vi "1_SimpleDemo_MHHisto.vi"() -> ()   [LabVIEW 2010]
uses:
  _lib/PQ/MultiHarp/mhlib_x86_x64_UIThread.llb/MH_DllPath_global.vi
  _lib/PQ/MultiHarp/MH_RefSource.ctl
  _lib/PQ/MultiHarp/MH_LibVersion_global.vi
  _lib/PQ/MultiHarp/MH_MeasMode.ctl
panel:
  in  "EnableInputDeadTime":bool caption="Enable DeadTime"
  in  "InputDeadTime":i32=1000 caption="DeadTime [ps]" min=800 max=160000 step=1
  in  "Trg.Edge":i32(ring) items=["falling", "rising"]
  in  "Trg.Level":i32=-100 caption="Trg.Level [mV]" min=-1200 max=1200 step=1
  in  "Offset":i32 caption="Offset [ps]" min=-99999 max=99999 step=1
  in  "Enable":bool=TRUE
  in  "EnableSyncDeadTime":bool caption="Enable DeadTime"
  in  "SyncDeadTime":i32=1000 caption="SyncDeadTime [ps]" min=800 max=160000 step=1
  in  "SyncTrg.Edge":i32(ring) items=["falling", "rising"]
  in  "SyncTrg.Level":i32=-100 caption="SyncTrg.Level [mV]" min=-1200 max=1200 step=1
  in  "SyncOffset":i32 caption="SyncOffset [ps]" min=-99999 max=99999 step=1
  in  "SyncDivider":i32(ring)=1 items=["1"=1, "2"=2, "4"=4, "8"=8, "16"=16]
  in  "Binning":i32(ring) caption="Resolution [ps]" items=["5", "10", "20", "40", "80", "160", "320", "640", "1280", "2560", "5120", "10240", "20480", "40960", "81920", "163840", "327680", "655360", "1310720", "2621440", "5242880", "10485760", "20971520", "41943040"]
  in  "HistoLength":i32(ring)=6 caption="Histo Length" items=["1024", "2048", "4096", "8192", "16384", "32768", "65536"]
  in  "Acqu.Time":i32=10000 caption="Acqu.Time [ms]" min=1 max=360000 step=1
  in  "GlobalOffset":i32 caption="GlobalOffset [ns]" min=0 max=100000000 step=1
  in  "OverflowLevel":u32=4294967295 min=1 step=1
  in  "StopOnOverflow":bool=TRUE
  out "HistoGraph":T1(graph)={0.0, "Resolution"=0.08, "Histogram"=array8x65536[524288 elements]}
  out "CountRates":i32[](array[numeric]) caption="Count Rates [cps]"
  out "SyncRate":i32 caption="Sync Rate [cps]"
  in  "stop":bool
  out "error out":errorcluster
  # "All Channels"
  # "Sync"
  # "Acquisition"
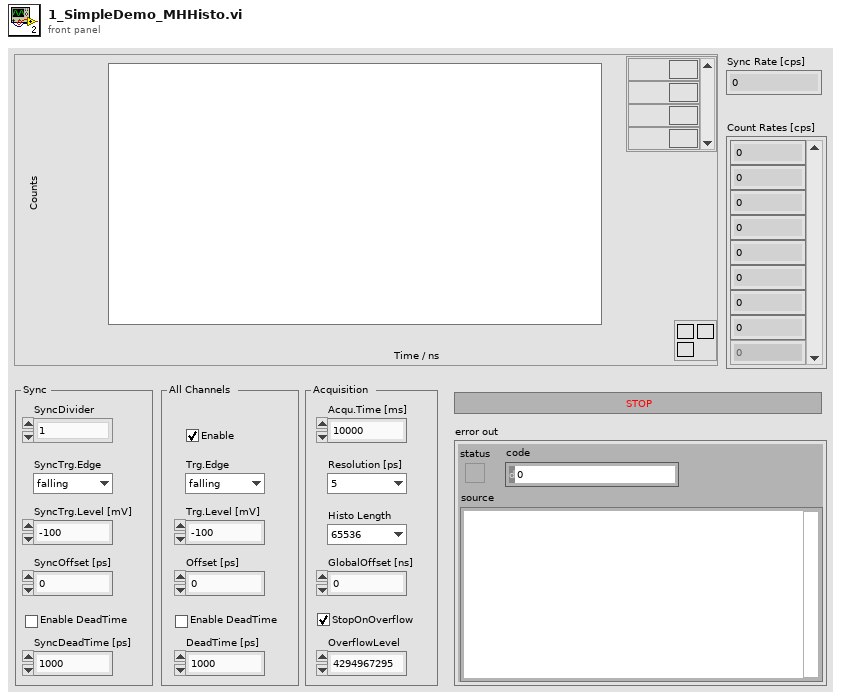
[diagram p1: front panel]
types:
  T1 = cluster{dbl, "Resolution":dbl, "Histogram":u32[][]}
  T2 = typedef "MH_MeasMode.ctl" = i32
  T3 = typedef "MH_RefSource.ctl" = enum16{"INTERNAL", "EXTERNAL_10MHZ", "WR_MASTER_GENERIC", "WR_SLAVE_GENERIC", "WR_GRANDM_GENERIC", "EXTN_GPS_PPS", "EXTN_GPS_PPS_UART", "WR_MASTER_MHARP", "WR_SLAVE_MHARP", "WR_GRANDM_MHARP"}
  T4 = typedef "MH_InitInfo.ctl" = cluster{"Library Version":string, "Serial No.":string, "Model":string, "Partnum":string, "Version":string, "features":i32, "nchannels":i32, "Base Resolution":dbl, "Bin Steps":i32}
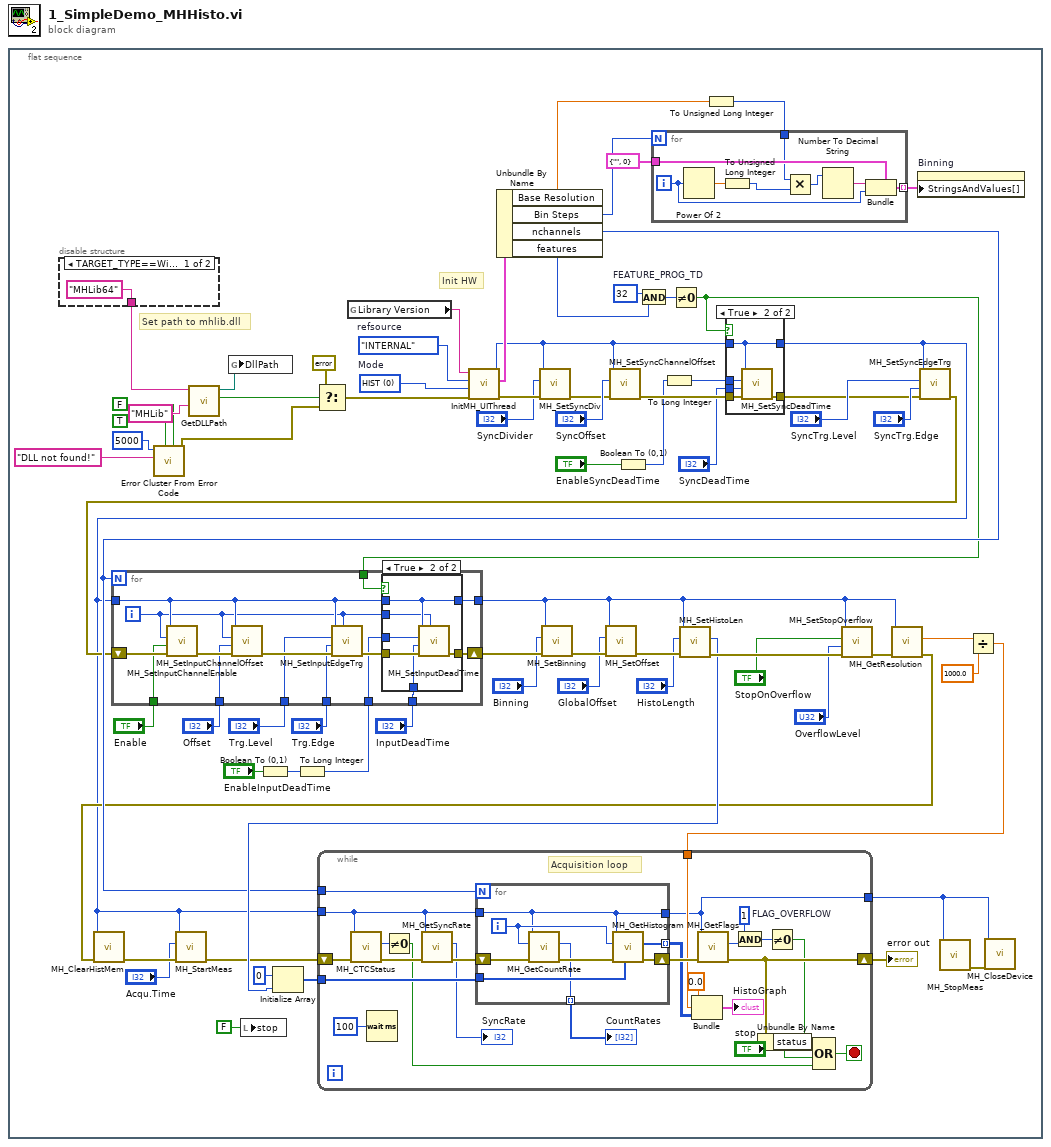
[diagram p0: block diagram]
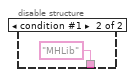
[diagram p3: hidden frame]
diagram:
  n1 = flat-sequence {
    frame #0 {
      w16 = 32  # FEATURE_PROG_TD
      w27 = T2 0 items=["HIST"=0, "T2"=2, "T3"=3]  # Mode
      w73 = MH_RefSource."INTERNAL"  # refsource
      # "Init HW"
      # "Set path to mhlib.dll"
      n2 = disable-structure shown="TARGET_TYPE==Windows, Default" {
        disable-tunnel: ["MHLib64" ("name or relative path") "MHLib" ("name or relative path")] -> w26
        frame condition #0 (active) {
        }
        frame condition #1 {
        }
      }
      n3 = call <vilib>:"Error Cluster From Error Code.vi"("is warning? (False)"=FALSE, "show call chain? (False)"=TRUE, "error message (\"\")"="DLL not found!" ("error message (\"\")"), "error code (0)"=5000) -> ("error out"=w72:errorcluster)  [unwired: 5 in]
      n4 = call "GetDLLPath.vi"("DllName_32bit"="MHLib" ("name or relative path"), "DllName_64bit"=w26) -> ("file exists?"=w70:bool, "DLLPath"=w69:path)  [unwired: 8 in]
      n5 = global write "MH_DllPath_global.vi" "DllPath"(w69) -> ()
      n6 = local write "stop"(FALSE ("stop")) -> ()
      n7 = Boolean To (0,1)(Boolean="EnableInputDeadTime") -> (0, 1=w12:i16)
      n8 = To Long Integer(number=w12) -> (32bit integer=w11:i32)
      n9 = Select(t=errorcluster {"status"=FALSE, "code"=0, "source"=""} ("error IO"), s=w70, f=w72) -> (s? t:f=w67:errorcluster)
      n10 = global read "MH_LibVersion_global.vi" "Library Version"() -> (w30:string)
      n11 = call "InitMH_UIThread.vi"("error in (no error)"=w67, "Mode"=w27, "refsource"=w73, "Library Version"=w30) -> ("error out"=w62:errorcluster, "Init Info"=w64:T4, "DevIdx"=w23:i32)  [unwired: 5 in]
      n12 = Unbundle By Name(w64) -> ("Base Resolution"=w7:dbl, "Bin Steps"=w8:i32, "nchannels"=w44:i32, "features"=w18:i32)
      n13 = call "MH_SetSyncDiv.vi"("error in (no error)"=w62, "SyncDivider"="SyncDivider", "devidx"=w23) -> ("error out"=w61:errorcluster)  [unwired: 7 in, 1 out]
      n14 = call "MH_SetSyncChannelOffset.vi"("error in (no error)"=w61, "Offset"="SyncOffset", "devidx"=w23) -> ("error out"=w25:errorcluster)  [unwired: 7 in, 1 out]
      n15 = Boolean To (0,1)(Boolean="EnableSyncDeadTime") -> (0, 1=w21:i16)
      n16 = And(x=w16, y=w18) -> (x .and. y?=w17:i32)
      n17 = To Long Integer(number=w21) -> (32bit integer=w20:i32)
      n18 = Not Equal To 0?(x=w17) -> (x != 0?=w10:bool)
      n19 = To Unsigned Long Integer(number=w7) -> (unsigned 32bit integer=w6:u32)
      n20 = for {
        N: w8 -> [_]
        tunnel: cluster{"String":string, "Value":i32} {"String"="", "Value"=0} -> [w81]
        tunnel: [w75] -> w5 mode=indexing
        tunnel: w6 -> [w74]
        i -> [w80]
        n21 = Power Of 2(x=w80) -> (2^x=w79:dbl)
        n22 = To Unsigned Long Integer(number=w79) -> (unsigned 32bit integer=w78:u32)
        n23 = Multiply(x=w74, y=w78) -> (x*y=w77:u32)
        n24 = Number To Decimal String(number=w77) -> (decimal integer string=w76:string)  [unwired: 1 in]
        n25 = Bundle(cluster=w81, "String"=w76, "Value"=w80) -> (w75:cluster{"String":string, "Value":i32})
      }
      n26 = case shown="True" w10 {
        tunnel: w25 -> [w82 w88]
        tunnel: [w82 w87] -> w24
        tunnel: w23 -> [w83 w84]
        tunnel: w20 -> [_ w86]
        tunnel: "SyncDeadTime" -> [_ w85]
        tunnel: [w83 w84] -> w15
        frame False {
        }
        frame True {
          n27 = call "MH_SetSyncDeadTime.vi"("error in (no error)"=w88, "deadtime"=w85, "on"=w86, "devidx"=w84) -> ("error out"=w87:errorcluster)  [unwired: 6 in, 1 out]
        }
      }
      n28 = property on="Binning" class="Ring (strict)"("StringsAndValues[]"=w5) -> ()  [unwired: 2 in, 2 out]
      n29 = call "MH_SetSyncEdgeTrg.vi"("error in (no error)"=w24, "edge"="SyncTrg.Edge", "level"="SyncTrg.Level", "devidx"=w15) -> ("error out"=w43:errorcluster)  [unwired: 6 in, 1 out]
      n30 = for {
        N: w44 -> [_]
        shift-right: [w129] -> w63
        shift-left: w43 -> [w138]
        tunnel: w15 -> [w130]
        tunnel: [w128] -> w38
        tunnel: "Enable" -> [w135]
        tunnel: "Offset" -> [w134]
        tunnel: "Trg.Edge" -> [w133]
        tunnel: "Trg.Level" -> [w132]
        tunnel: "InputDeadTime" -> [w126]
        tunnel: w11 -> [w125]
        tunnel: w10 -> [w124]
        i -> [w127]
        n31 = call "MH_SetInputChannelEnable.vi"("error in (no error)"=w138, "enable"=w135, "channel"=w127, "devidx"=w130) -> ("error out"=w137:errorcluster)  [unwired: 6 in, 1 out]
        n32 = call "MH_SetInputChannelOffset.vi"("error in (no error)"=w137, "Offset"=w134, "channel"=w127, "devidx"=w130) -> ("error out"=w136:errorcluster)  [unwired: 6 in, 1 out]
        n33 = call "MH_SetInputEdgeTrg.vi"("channel"=w127, "error in (no error)"=w136, "edge"=w133, "level"=w132, "devidx"=w130) -> ("error out"=w131:errorcluster)  [unwired: 5 in, 1 out]
        n34 = case shown="True" w124 {
          tunnel: w131 -> [w140 w146]
          tunnel: w130 -> [w139 w144]
          tunnel: [w140 w145] -> w129
          tunnel: [w139 w144] -> w128
          tunnel: w127 -> [_ w143]
          tunnel: w126 -> [_ w142]
          tunnel: w125 -> [_ w141]
          frame False {
          }
          frame True {
            n35 = call "MH_SetInputDeadTime.vi"("channel"=w143, "error in (no error)"=w146, "deadtime"=w142, "on"=w141, "devidx"=w144) -> ("error out"=w145:errorcluster)  [unwired: 5 in, 1 out]
          }
        }
      }
      n36 = call "MH_SetBinning.vi"("error in (no error)"=w63, "Binning"="Binning", "devidx"=w38) -> ("error out"=w59:errorcluster)  [unwired: 7 in, 1 out]
      n37 = call "MH_SetOffset.vi"("error in (no error)"=w59, "Offset"="GlobalOffset", "devidx"=w38) -> ("error out"=w57:errorcluster)  [unwired: 7 in, 1 out]
      n38 = call "MH_SetHistoLen.vi"("error in (no error)"=w57, "lencode"="HistoLength", "devidx"=w38) -> ("error out"=w56:errorcluster, "actuallen"=w49:i32)  [unwired: 6 in, 1 out]
      n39 = Initialize Array(u32 0, w49) -> (w48:u32[])
      n40 = call "MH_SetStopOverflow.vi"("error in (no error)"=w56, "stopcount"="OverflowLevel", "StopOnOverflow"="StopOnOverflow", "devidx"=w38) -> ("error out"=w39:errorcluster)  [unwired: 6 in, 1 out]
      n41 = call "MH_GetResolution.vi"("error in (no error)"=w39, "devidx"=w38) -> ("error out"=w36:errorcluster, "resolution"=w37:dbl)  [unwired: 7 in, 1 out]
      n42 = call "MH_ClearHistMem.vi"("error in (no error)"=w36, "devidx"=w15) -> ("error out"=w53:errorcluster)  [unwired: 8 in, 1 out]
      n43 = call "MH_StartMeas.vi"("error in (no error)"=w53, "tacq"="Acqu.Time", "devidx"=w15) -> ("error out"=w35:errorcluster)  [unwired: 7 in, 1 out]
      n44 = Divide(x=w37, y=1000.0) -> (x/y=w45:dbl)
      n45 = while {
        shift-right: [w103] -> w51
        shift-left: w35 -> [w114]
        tunnel: w15 -> [w110]
        tunnel: w44 -> [w113]
        tunnel: w48 -> [w105]
        tunnel: w45 -> [w97]
        tunnel: [w92] -> w29
        stop <- w104 stop-if-true
        w108 = 1  # FLAG_OVERFLOW
        # "Acquisition loop"
        n46 = call "MH_CTCStatus.vi"("error in (no error)"=w114, "devidx"=w110) -> ("error out"=w112:errorcluster, "ctcstatus"=w115:i32)  [unwired: 7 in, 1 out]
        n47 = Wait (ms)(milliseconds to wait=u32 100) -> ()  [unwired: 1 out]
        n48 = Not Equal To 0?(x=w115) -> (x != 0?=w94:bool)
        n49 = call "MH_GetSyncRate.vi"("error in (no error)"=w112, "devidx"=w110) -> ("error out"=w111:errorcluster, "syncrate"=→"SyncRate":i32)  [unwired: 7 in, 1 out]
        n50 = for {
          N: w113 -> [_]
          shift-right: [w123] -> w109
          shift-left: w111 -> [w122]
          tunnel: w110 -> [w119]
          tunnel: [w119] -> w92
          tunnel: w105 -> [w118]
          tunnel: [w117] -> w100 mode=indexing
          tunnel: [w116] -> w99 mode=indexing
          i -> [w120]
          n51 = call "MH_GetCountRate.vi"("error in (no error)"=w122, "Channel"=w120, "devidx"=w119) -> ("error out"=w121:errorcluster, "rate"=w117:i32)  [unwired: 6 in, 1 out]
          n52 = call "MH_GetHistogram.vi"("Chcount"=w118, "error in (no error)"=w121, "channel"=w120, "devidx"=w119) -> ("error out"=w123:errorcluster, "Histogram"=w116:u32[])  [unwired: 5 in, 1 out]
        }
        "CountRates" <- w100
        n53 = Bundle(0.0, w97, "Histogram"=w99) -> (→"HistoGraph":cluster{dbl, dbl, "Histogram":u32[][]})  [unwired: 1 in]
        n54 = call "MH_GetFlags.vi"("error in (no error)"=w109, "devidx"=w92) -> ("error out"=w103:errorcluster, "flags"=w106:i32)  [unwired: 7 in, 1 out]
        n55 = And(x=w108, y=w106) -> (x .and. y?=w107:i32)
        n56 = Unbundle By Name(w103) -> ("status"=w91:bool)
        n57 = Not Equal To 0?(x=w107) -> (x != 0?=w102:bool)
        n58 = Compound Arithmetic op=OR(w91, w102, "stop", w94) -> (w104:bool)
      }
      "error out" <- w51
      n59 = call "MH_StopMeas.vi"("devidx"=w29) -> ("error out"=w28:errorcluster)  [unwired: 9 in, 1 out]
      n60 = call "MH_CloseDevice.vi"("error in (no error)"=w28, "devidx"=w29) -> ()  [unwired: 8 in, 2 out]
    }
  }
